vi "UDPreciever-old.vi"() -> ()   [LabVIEW 2012]
panel:
  out "appended array 2":string[](array[string])
  out "channel":u32
  out "appended array":bool[][](array[boolean])
  out "Found Header 2":bool
  out "word 7":u8[](array[numeric]) format="%02x"
  out "word 6":u8[](array[numeric]) format="%02x"
  out "word 5":u8[](array[numeric]) format="%02x"
  out "word 4":u8[](array[numeric]) format="%02x"
  out "subarray":bool[](array[boolean])
  out "in 10":bool
  out "in 9":bool
  out "in 8":bool
  out "in 7":bool
  out "in 6":bool
  out "in 5":bool
  out "in 4":bool
  out "in 3":bool
  out "in 2":bool
  out "in 1":bool
  out "in 0":bool
  out "in 11":bool
  out "channel 11":u32[](graph)
  out "channel 10":u32[](graph)
  out "channel 9":u32[](graph)
  out "channel 8":u32[](graph)
  out "channel 7":u32[](graph)
  out "channel 6":u32[](graph)
  out "channel 5":u32[](graph)
  out "channel 4":u32[](graph)
  out "channel 3":u32[](graph)
  out "channel 2":u32[](graph)
  out "channel 1":u32[](graph)
  out "channel 0":u32[](graph)
  out "frameCntr":u32
  out "rTime":u32
  out "Channel":u32
  out "Sync":u32
  out "Prof/Hist":u32
  out "Cnts/Bin":u32
  out "NumBins":u32
  out "Found Header":bool
  out "MultiDimHeader":bool[][](array[boolean])
  out "i":i32
  out "word 0":u8[](array[numeric]) format="%02x"
  out "word 1":u8[](array[numeric]) format="%02x"
  out "word 2":u8[](array[numeric]) format="%02x"
  out "word 3":u8[](array[numeric]) format="%02x"
  out "First Element":string
  out "Raw Data Out":string
  out "error post-check":errorcluster
  out "End Reciever Error":errorcluster
  in  "stop reciever":bool
  out "port":u16
  out "error out post-read":errorcluster
  out "error out pre-read":errorcluster
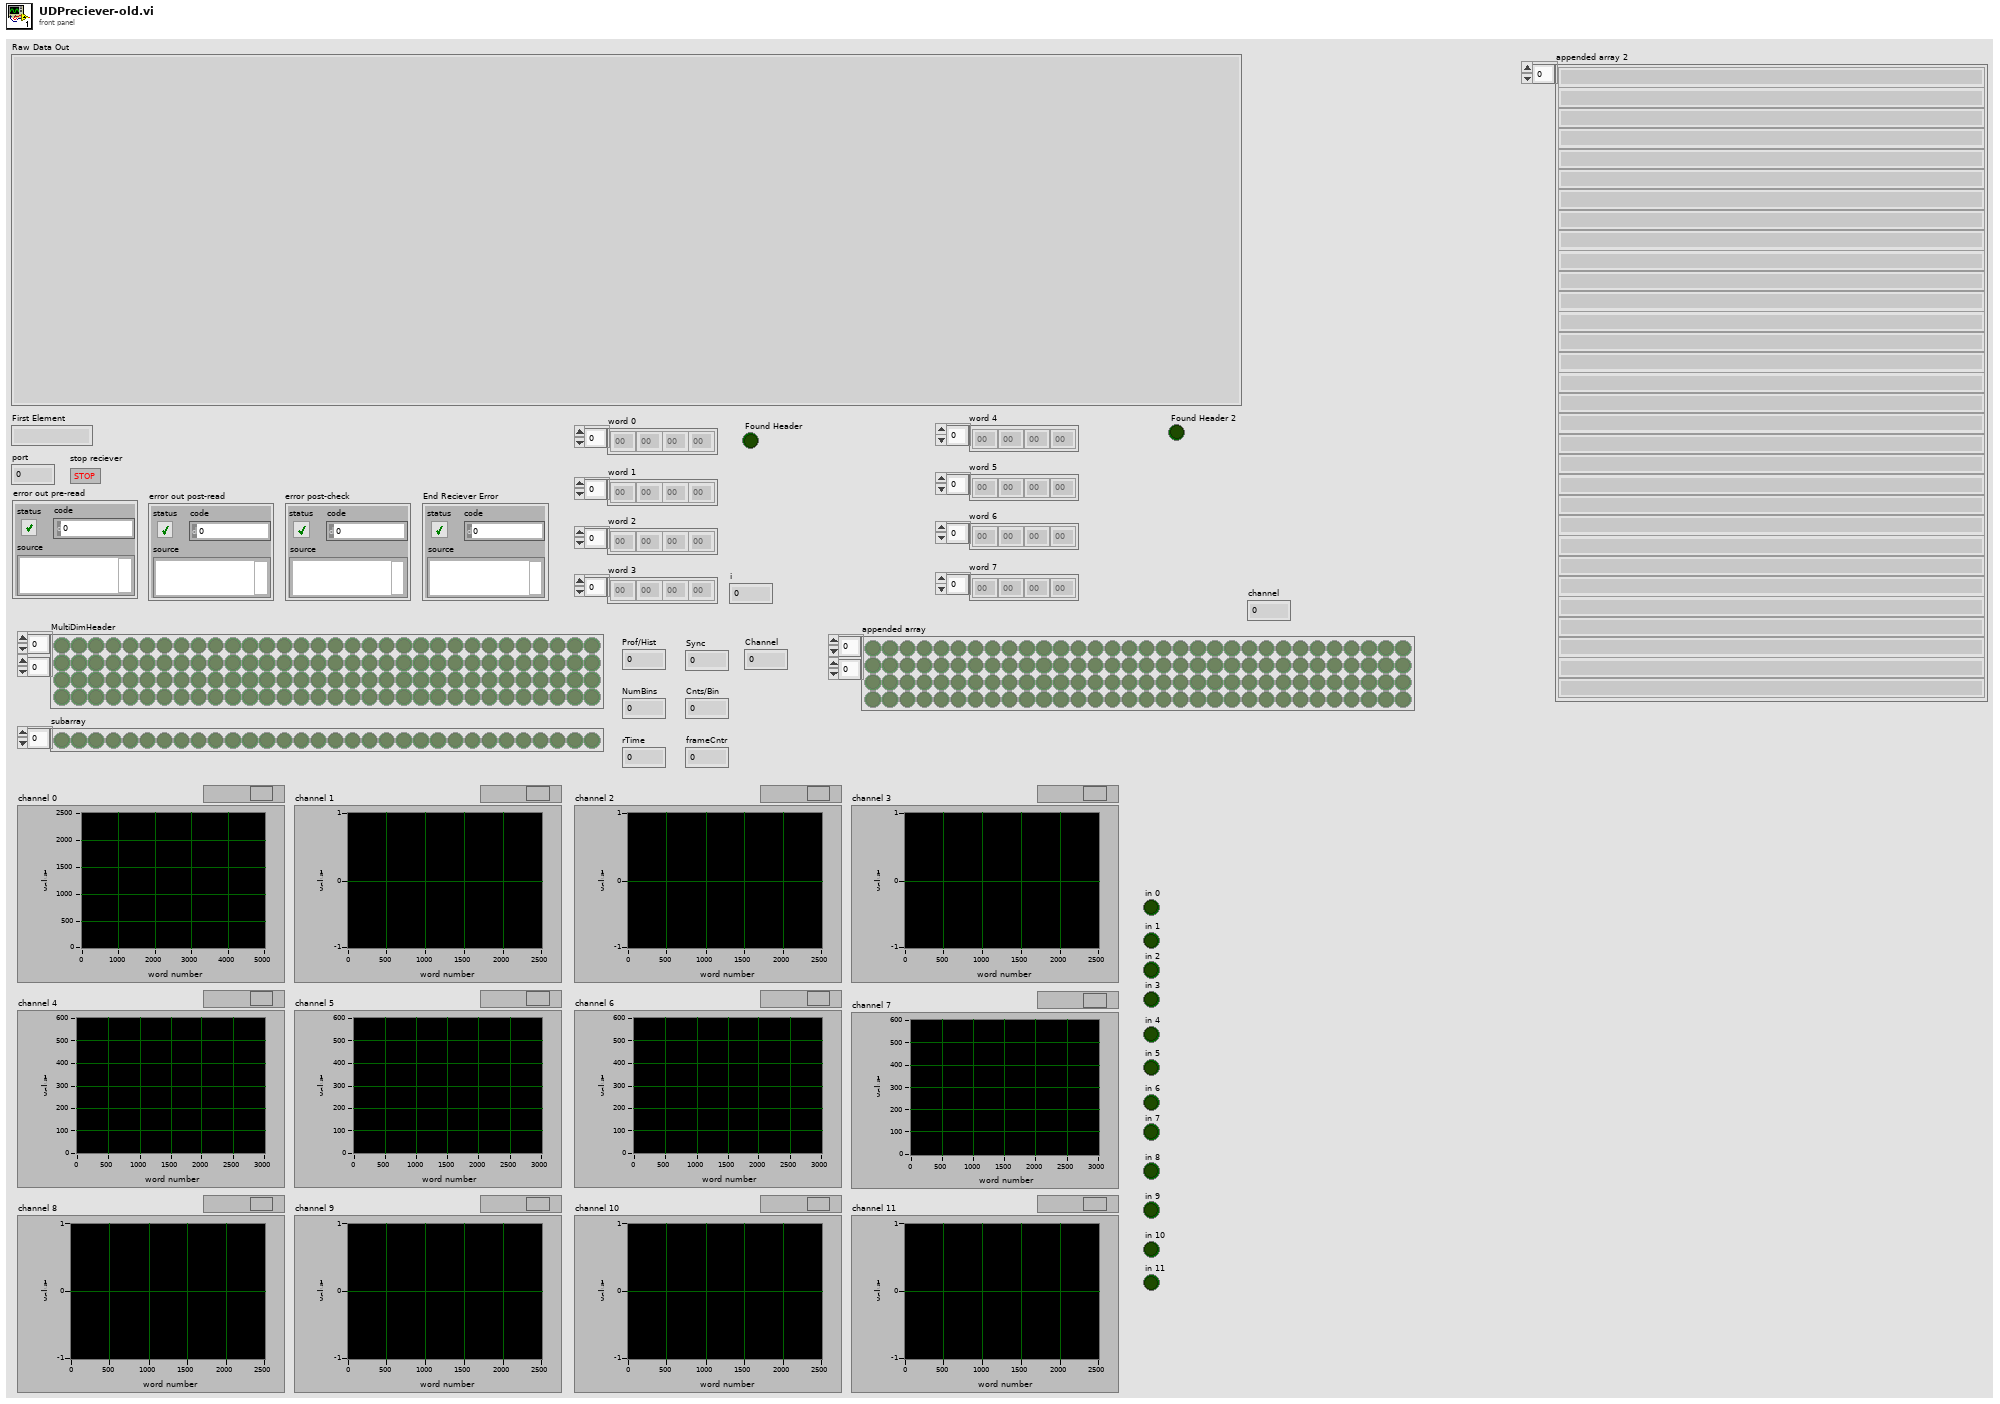
[diagram p1: front panel]
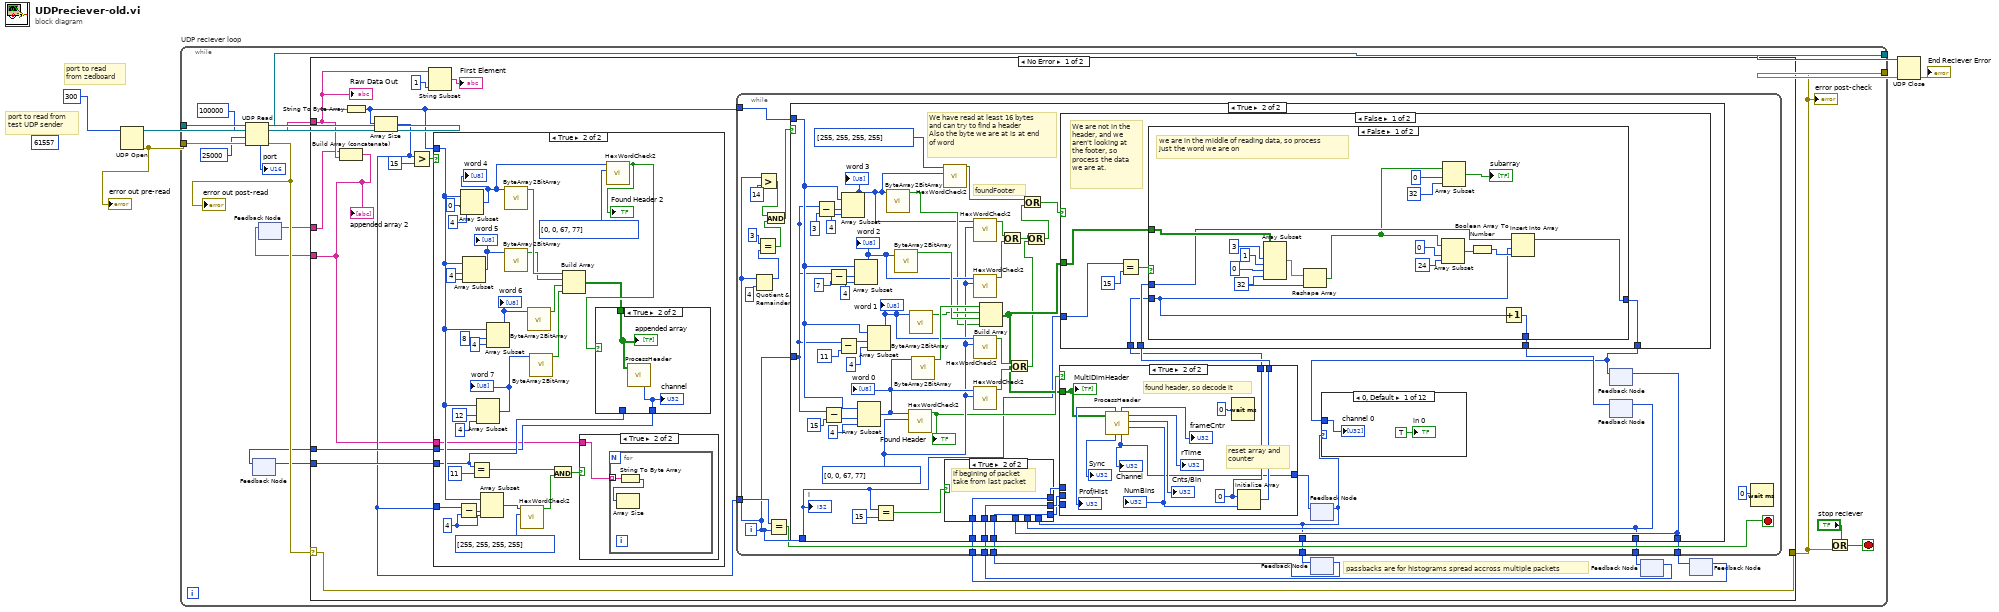
[diagram p0: block diagram]
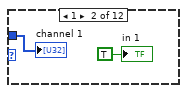
[diagram p6: hidden frame]
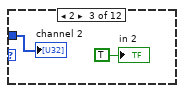
[diagram p7: hidden frame]
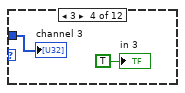
[diagram p8: hidden frame]
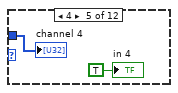
[diagram p9: hidden frame]
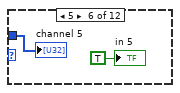
[diagram p10: hidden frame]
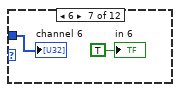
[diagram p11: hidden frame]
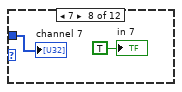
[diagram p12: hidden frame]
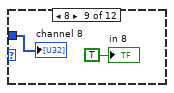
[diagram p13: hidden frame]
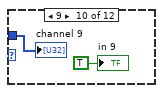
[diagram p14: hidden frame]
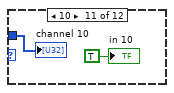
[diagram p15: hidden frame]
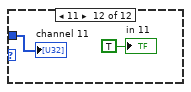
[diagram p16: hidden frame]
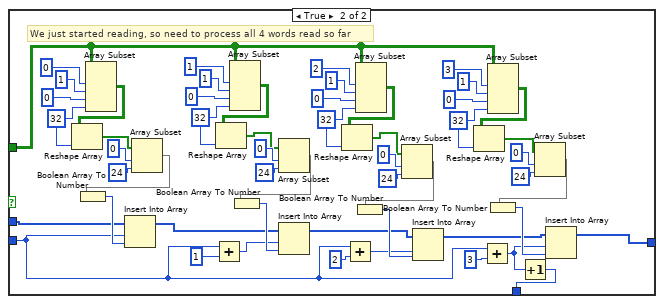
[diagram p18: hidden frame]
diagram:
  (unwired) u16 61557 ("port")
  # "port to read \nfrom zedboard"
  # "port to read from \ntest UDP sender"
  n1 = UDP Open(11:u16 300 ("port")) -> (port=w5:refnum<k16>, 0:w2:errorcluster)  [unwired: 4 in, 1 out]
  "error out pre-read" <- w2
  n2 = while "UDP reciever loop" {
    tunnel: [w21] -> w6
    tunnel: w5 -> [w20]
    tunnel: [w12] -> w4
    tunnel: w2 -> [w17]
    stop <- w19 stop-if-true
    n3 = UDP Read(connection ID=w20, max size (548)=100000, timeout ms (25000)=25000, 8:w17) -> (data out=w14:string, error out=w16:errorcluster, 3:w21:refnum<k16>, 4:→"port":u16)  [unwired: 1 out]
    "error out post-read" <- w16
    n4 = feedback #1() -> (w7:u32)  [unwired: 1 in]
    n5 = feedback #2() -> (w9:string[])  [unwired: 1 in]
    n6 = case shown="No Error" w16 {
      selector: w16 -> [w31 w279]
      tunnel: w14 -> [w30 _]
      tunnel: [w31 w279] -> w12
      tunnel: [w22 w278] -> w10
      tunnel: w9 -> [w29 w278]
      tunnel: [w25 w277] -> w8
      tunnel: w7 -> [w24 w277]
      frame No Error {
        # "passbacks are for histograms spread accross multiple packets"
        n7 = Build Array (concatenate)(w29, w30) -> (w22:string[])
        "appended array 2" <- w22
        n8 = String To Byte Array(string=w30) -> (unsigned byte array=w26:u8[])
        n9 = Array Size(array=w26) -> (size(s)=w23:i32)
        n10 = Greater?(x=w23, y=15) -> (0:w28:bool)
        n11 = String Subset(string=w30, length (rest)=1 ("length (rest)")) -> (substring=→"First Element":string)  [unwired: 1 in]
        n12 = case shown="True" w28 {
          tunnel: w26 -> [_ w48]
          tunnel: [w40 w42] -> w25
          tunnel: w24 -> [w40 w43]
          tunnel: w23 -> [_ w45]
          tunnel: w22 -> [_ w41]
          frame False {
          }
          frame True {
            w47 = 4 ("length")
            w66 = 4 ("length")
            n13 = Subtract(x=w45, y=w47) -> (x-y=w46:i32)
            n14 = Array Subset(array=w48, index=0, length=4) -> (w55:u8[])
            "word 4" <- w55
            n15 = Array Subset(array=w48, index=w66, length=w66) -> (w71:u8[])
            "word 5" <- w71
            n16 = Equal?(x=w43, y=u32 11) -> (x = y?=w50:bool)
            n17 = Array Subset(array=w48, index=12, length=4) -> (w53:u8[])
            "word 7" <- w53
            n18 = Array Subset(array=w48, index=w46, length=w47) -> (w44:u8[])
            n19 = Array Subset(array=w48, index=8, length=4) -> (w70:u8[])
            "word 6" <- w70
            n20 = call "ByteArray2BitArray.vi"("array"=w55) -> ("Array"=w61:bool[])  [unwired: 10 in]
            n21 = call "ByteArray2BitArray.vi"("array"=w71) -> ("Array"=w60:bool[])  [unwired: 10 in]
            n22 = call "HexWordCheck2.vi"("array"=u8[] [255, 255, 255, 255], "Input Array"=w44) -> ("Boolean"=w49:bool)  [unwired: 9 in]
            n23 = call "ByteArray2BitArray.vi"("array"=w70) -> ("Array"=w58:bool[])  [unwired: 10 in]
            n24 = call "ByteArray2BitArray.vi"("array"=w53) -> ("Array"=w59:bool[])  [unwired: 10 in]
            n25 = And(x=w50, y=w49) -> (x .and. y?=w52:bool)
            n26 = Build Array(w61, w60, w58, w59) -> (w56:bool[][])
            n27 = case shown="True" w52 {
              tunnel: w41 -> [_ w72]
              frame False {
              }
              frame True {
                n28 = for {
                  tunnel: w72 -> [w74] mode=indexing
                  n29 = String To Byte Array(string=w74) -> (unsigned byte array=w73:u8[])
                  n30 = Array Size(array=w73) -> ()  [unwired: 1 out]
                }
              }
            }
            n31 = call "HexWordCheck2.vi"("array"=u8[] [0, 0, 67, 77], "Input Array"=w55) -> ("Boolean"=w57:bool)  [unwired: 9 in]
            "Found Header 2" <- w57
            n32 = case shown="True" w57 {
              tunnel: w56 -> [_ w77]
              tunnel: [w75 w76] -> w42
              tunnel: w43 -> [w75 _]
              frame False {
              }
              frame True {
                n33 = call "ProcessHeader.vi"("Array"=w77) -> ("Numeric 4"=w76:u32)  [unwired: 4 in, 6 out]
                "channel" <- w76
                "appended array" <- w77
              }
            }
          }
        }
        n34 = feedback #3() -> (w32:u32)  [unwired: 1 in]
        n35 = feedback #4() -> (w34:u32)  [unwired: 1 in]
        n36 = feedback #5() -> (w35:u32[])  [unwired: 1 in]
        n37 = while {
          tunnel: w26 -> [w92]
          tunnel: w23 -> [w95]
          tunnel: [w83] -> w37
          tunnel: [w82] -> w36
          tunnel: w35 -> [w81]
          tunnel: w34 -> [w80]
          tunnel: [w79] -> w33
          tunnel: w32 -> [w78]
          i -> [w91]
          stop <- w84 stop-if-true
          n38 = Quotient & Remainder(x=w91, y=4) -> (x-y*floor(x/y)=w89:i32)  [unwired: 1 out]
          n39 = Equal?(x=3, y=w89) -> (x = y?=w85:bool)
          n40 = Greater?(x=w91, y=14 ("x")) -> (0:w87:bool)
          n41 = And(x=w87, y=w85) -> (x .and. y?=w86:bool)
          n42 = Equal?(x=w95, y=w91) -> (x = y?=w84:bool)
          n43 = case shown="True" w86 {
            tunnel: w92 -> [_ w135]
            tunnel: w91 -> [_ w134]
            tunnel: w91 -> [_ w109]
            tunnel: [w98 w112] -> w83
            tunnel: [w97 w105] -> w82
            tunnel: w81 -> [w98 w114]
            tunnel: w80 -> [w97 w113]
            tunnel: [w96 w100] -> w79
            tunnel: w78 -> [w96 w103]
            frame False {
            }
            frame True {
              w124 = u8[] [0, 0, 67, 77] ("array")
              # "foundFooter"
              # "We have read at least 16 bytes \nand can try to find a header\nAlso the byte we are at is at end \nof word"
              n44 = Subtract(x=w134, y=3) -> (x-y=w150:i32)
              n45 = Subtract(x=w134, y=15) -> (x-y=w144:i32)
              n46 = Subtract(x=w134, y=7) -> (x-y=w148:i32)
              n47 = Subtract(x=w134, y=11) -> (x-y=w146:i32)
              n48 = Array Subset(array=w135, index=w150, length=4) -> (w119:u8[])
              "word 3" <- w119
              n49 = Array Subset(array=w135, index=w148, length=4) -> (w133:u8[])
              "word 2" <- w133
              n50 = Array Subset(array=w135, index=w144, length=4) -> (w126:u8[])
              "word 0" <- w126
              n51 = Array Subset(array=w135, index=w146, length=4) -> (w132:u8[])
              "word 1" <- w132
              n52 = Equal?(x=w109, y=15) -> (x = y?=w107:bool)
              n53 = call "ByteArray2BitArray.vi"("array"=w119) -> ("Array"=w121:bool[])  [unwired: 10 in]
              n54 = call "ByteArray2BitArray.vi"("array"=w133) -> ("Array"=w137:bool[])  [unwired: 10 in]
              n55 = call "HexWordCheck2.vi"("array"=w124, "Input Array"=w126) -> ("Boolean"=w123:bool)  [unwired: 9 in]
              "Found Header" <- w123
              n56 = call "ByteArray2BitArray.vi"("array"=w132) -> ("Array"=w136:bool[])  [unwired: 10 in]
              n57 = call "ByteArray2BitArray.vi"("array"=w126) -> ("Array"=w138:bool[])  [unwired: 10 in]
              n58 = call "HexWordCheck2.vi"("array"=w119, "Input Array"=u8[] [255, 255, 255, 255] ("array")) -> ("Boolean"=w104:bool)  [unwired: 9 in]
              n59 = call "HexWordCheck2.vi"("array"=w124, "Input Array"=w119) -> ("Boolean"=w129:bool)  [unwired: 9 in]
              n60 = call "HexWordCheck2.vi"("array"=w124, "Input Array"=w133) -> ("Boolean"=w128:bool)  [unwired: 9 in]
              n61 = call "HexWordCheck2.vi"("array"=w124, "Input Array"=w132) -> ("Boolean"=w130:bool)  [unwired: 9 in]
              n62 = call "HexWordCheck2.vi"("array"=w124, "Input Array"=w126) -> ("Boolean"=w131:bool)  [unwired: 9 in]
              n63 = Build Array(w138, w136, w137, w121) -> (w122:bool[][])
              n64 = Or(x=w129, y=w128) -> (x .or. y?=w127:bool)
              n65 = Or(x=w130, y=w131) -> (x .or. y?=w115:bool)
              n66 = Or(x=w127, y=w115) -> (x .or. y?=w118:bool)
              n67 = Or(x=w104, y=w118) -> (x .or. y?=w117:bool)
              n68 = feedback #6() -> (w100:u32)  [unwired: 1 in]
              n69 = feedback #7() -> (w112:u32[])  [unwired: 1 in]
              n70 = feedback #8() -> (w105:u32)  [unwired: 1 in]
              n71 = case shown="True" w107 {
                tunnel: w114 -> [_ w180]
                tunnel: w113 -> [_ w179]
                tunnel: w105 -> [w176 _]
                tunnel: w112 -> [w177 _]
                tunnel: [w176 w179] -> w111
                tunnel: [w177 w180] -> w110
                tunnel: w103 -> [_ w178]
                tunnel: [w175 w178] -> w102
                tunnel: w100 -> [w175 _]
                frame False {
                  # "if middle of packet\ntake from this loop"
                }
                frame True {
                  # "if begining of packet\ntake from last packet"
                }
              }
              n72 = case shown="True" w123 {
                tunnel: w122 -> [_ w272]
                tunnel: [w264 w269] -> w125
                tunnel: [w265 w267] -> w116
                tunnel: w111 -> [w265 _]
                tunnel: w110 -> [w264 _]
                tunnel: [w263 w266] -> w101
                tunnel: w102 -> [w263 _]
                frame False {
                  # "didn't find header so keep info from \nlast itteration of loop"
                }
                frame True {
                  w267 = u32 0 ("element")
                  # "reset array and \ncounter"
                  # "found header, so decode it"
                  n73 = call "ProcessHeader.vi"("Array"=w272) -> ("Numeric"=w268:u32, "Numeric 7"=→"Cnts/Bin":u32, "Numeric 3"=→"rTime":u32, "Numeric 4"=w266:u32, "Numeric 2"=→"frameCntr":u32, "Numeric 5"=→"Sync":u32, "Numeric 6"=→"Prof/Hist":u32)  [unwired: 4 in]
                  "NumBins" <- w268
                  "Channel" <- w266
                  n74 = Wait (ms)(milliseconds to wait=u32 0) -> ()  [unwired: 1 out]
                  n75 = Initialize Array(w267, w268) -> (w269:u32[])
                  "MultiDimHeader" <- w272
                }
              }
              n76 = case shown="False" w117 {
                tunnel: w109 -> [w183 _]
                tunnel: w125 -> [w184 w262]
                tunnel: [w185 w262] -> w99
                tunnel: w122 -> [w186 _]
                tunnel: w116 -> [w182 w261]
                tunnel: [w181 w261] -> w106
                frame False {
                  # "We are not in the \nheader, and we \naren't looking at \nthe footer, so \nprocess the data \nwe are at."
                  n77 = Equal?(x=w183, y=15) -> (x = y?=w187:bool)
                  n78 = case shown="False" w187 {
                    tunnel: w186 -> [w197 w240]
                    tunnel: [w195 w215] -> w185
                    tunnel: w184 -> [w196 w234]
                    tunnel: w182 -> [w193 w212]
                    tunnel: [w194 w208] -> w181
                    frame False {
                      w206 = 32 ("length")
                      # "we are in the middle of reading data, so process \njust the word we are on"
                      n79 = Array Subset(array=w197, index (row)=3 ("index"), length (row)=1 ("length"), index (col)=0 ("index"), length (col)=w206) -> (w205:bool[][])
                      n80 = Reshape Array(w205, w206) -> (w192:bool[])
                      n81 = Array Subset(array=w192, index=0, length=24) -> (w198:bool[])
                      n82 = Array Subset(array=w192, index=0, length=32) -> (→"subarray":bool[])
                      n83 = Boolean Array To Number(Boolean array=w198) -> (number=w201:u32)
                      n84 = Increment(x=w193) -> (x+1=w194:u32)
                      n85 = Insert Into Array(array=w196, index=w193, new element=w201) -> (w195:u32[])
                    }
                    frame True {
                      w242 = 32 ("length")
                      w247 = 32 ("length")
                      w252 = 32 ("length")
                      w257 = 32 ("length")
                      # "We just started reading, so need to process all 4 words read so far"
                      n86 = Array Subset(array=w240, index (row)=0 ("index"), length (row)=1 ("length"), index (col)=0 ("index"), length (col)=w257) -> (w256:bool[][])
                      n87 = Reshape Array(w256, w257) -> (w235:bool[])
                      n88 = Array Subset(array=w235, index=0, length=24) -> (w239:bool[])
                      n89 = Boolean Array To Number(Boolean array=w239) -> (number=w236:u32)
                      n90 = Insert Into Array(array=w234, index=w212, new element=w236) -> (w228:u32[])
                      n91 = Add(x=w212, y=u32 1) -> (x+y=w213:u32)
                      n92 = Array Subset(array=w240, index (row)=1 ("index"), length (row)=1 ("length"), index (col)=0 ("index"), length (col)=w252) -> (w251:bool[][])
                      n93 = Reshape Array(w251, w252) -> (w231:bool[])
                      n94 = Array Subset(array=w231, index=0, length=24) -> (w229:bool[])
                      n95 = Boolean Array To Number(Boolean array=w229) -> (number=w230:u32)
                      n96 = Insert Into Array(array=w228, index=w213, new element=w230) -> (w222:u32[])
                      n97 = Add(x=w212, y=u32 2) -> (x+y=w214:u32)
                      n98 = Array Subset(array=w240, index (row)=2 ("index"), length (row)=1 ("length"), index (col)=0 ("index"), length (col)=w247) -> (w246:bool[][])
                      n99 = Reshape Array(w246, w247) -> (w224:bool[])
                      n100 = Array Subset(array=w224, index=0, length=24) -> (w223:bool[])
                      n101 = Boolean Array To Number(Boolean array=w223) -> (number=w225:u32)
                      n102 = Insert Into Array(array=w222, index=w214, new element=w225) -> (w216:u32[])
                      n103 = Add(x=w212, y=u32 3) -> (x+y=w207:u32)
                      n104 = Array Subset(array=w240, index (row)=3 ("index"), length (row)=1 ("length"), index (col)=0 ("index"), length (col)=w242) -> (w241:bool[][])
                      n105 = Reshape Array(w241, w242) -> (w218:bool[])
                      n106 = Increment(x=w207) -> (x+1=w208:u32)
                      n107 = Array Subset(array=w218, index=0, length=24) -> (w217:bool[])
                      n108 = Boolean Array To Number(Boolean array=w217) -> (number=w219:u32)
                      n109 = Insert Into Array(array=w216, index=w207, new element=w219) -> (w215:u32[])
                    }
                  }
                }
                frame True {
                }
              }
              n110 = feedback-in #6(w101) -> ()
              n111 = case shown="0, Default" w100 {
                tunnel: w99 -> [w152 w154 w156 w158 w160 w162 w164 w166 w168 w170 w172 w174]
                frame 0, Default {
                  "channel 0" <- w152
                  "in 0" <- TRUE ("in 11")
                }
                frame 1 {
                  "channel 1" <- w154
                  "in 1" <- TRUE ("in 11")
                }
                frame 2 {
                  "channel 2" <- w156
                  "in 2" <- TRUE ("in 11")
                }
                frame 3 {
                  "channel 3" <- w158
                  "in 3" <- TRUE ("in 11")
                }
                frame 4 {
                  "channel 4" <- w160
                  "in 4" <- TRUE ("in 11")
                }
                frame 5 {
                  "channel 5" <- w162
                  "in 5" <- TRUE ("in 11")
                }
                frame 6 {
                  "channel 6" <- w164
                  "in 6" <- TRUE ("in 11")
                }
                frame 7 {
                  "channel 7" <- w166
                  "in 7" <- TRUE ("in 11")
                }
                frame 8 {
                  "channel 8" <- w168
                  "in 8" <- TRUE ("in 11")
                }
                frame 9 {
                  "channel 9" <- w170
                  "in 9" <- TRUE ("in 11")
                }
                frame 10 {
                  "channel 10" <- w172
                  "in 10" <- TRUE ("in 11")
                }
                frame 11 {
                  "channel 11" <- w174
                  "in 11" <- TRUE ("in 11")
                }
              }
              n112 = feedback-in #7(w99) -> ()
              n113 = feedback-in #8(w106) -> ()
              "i" <- w109
            }
          }
          n114 = Wait (ms)(milliseconds to wait=u32 0) -> ()  [unwired: 1 out]
        }
        n115 = feedback-in #3(w33) -> ()
        n116 = feedback-in #4(w36) -> ()
        n117 = feedback-in #5(w37) -> ()
        "Raw Data Out" <- w30
      }
      frame Error {
      }
    }
    "error post-check" <- w12
    n118 = feedback-in #1(w8) -> ()
    n119 = feedback-in #2(w10) -> ()
    n120 = Or(x="stop reciever", y=w12) -> (x .or. y?=w19:bool)
  }
  n121 = UDP Close(connection ID=w6, 8:w4) -> (error out=→"End Reciever Error":errorcluster)  [unwired: 1 out]
